vi "get hdf label list swig.vi"(9 "nDevices":i32, 10 "monitor_labels":T1, 11 "file":string) -> (1 "nDevices out":i32, 2 "monitor_labels out":T1, 3 "file out":string, 5 "function return":i32)   [LabVIEW 2019, in "apdm.lvlib"]
doc: "APDM_EXPORT int apdm_get_hdf_label_list_swig(char *file, apdm_monitor_label_t *monitor_labels, int *nDevices);"
uses:
  apdm.lvlib
  Lee Lab/CP FES Walking 2018/Code/Working/LabVIEW/apdm.dll
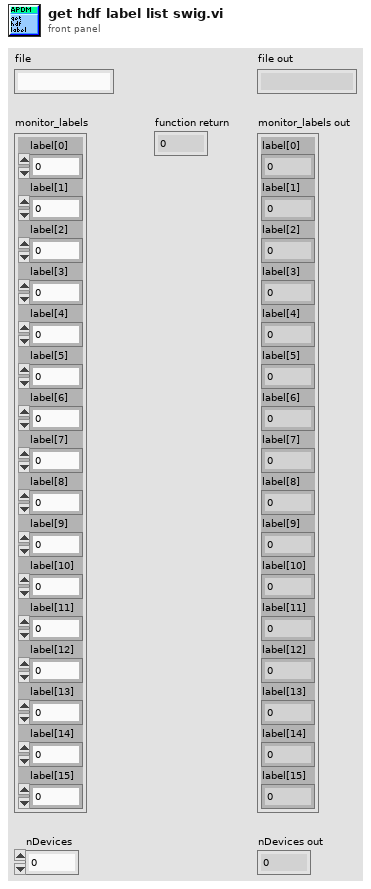
[diagram p1: front panel]
types:
  T1 = cluster{"label[0]":i8, "label[1]":i8, "label[2]":i8, "label[3]":i8, "label[4]":i8, "label[5]":i8, "label[6]":i8, "label[7]":i8, "label[8]":i8, "label[9]":i8, "label[10]":i8, "label[11]":i8, "label[12]":i8, "label[13]":i8, "label[14]":i8, "label[15]":i8}
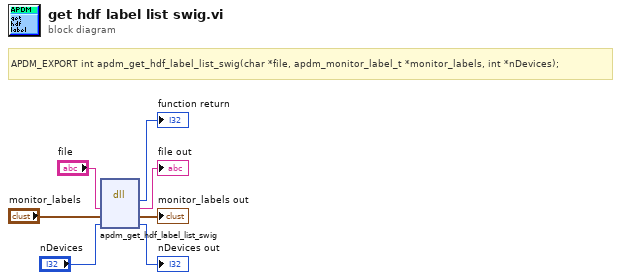
[diagram p0: block diagram]
diagram:
  # "APDM_EXPORT\tint apdm_get_hdf_label_list_swig(char *file, apdm_monitor_label_t *monitor_labels, int *nDevices);"
  n1 = dll-call lib="C:/Users/jfalesi/Dropbox/Lee Lab/CP FES Walking 2018/Code/Working/LabVIEW/apdm.*" fn="apdm_get_hdf_label_list_swig"("file"="file", "monitor_labels"="monitor_labels", "nDevices"="nDevices") -> (→"function return":i32, "file"=→"file out":string, "monitor_labels"=→"monitor_labels out":T1, "nDevices"=→"nDevices out":i32)  [unwired: 3 in, 2 out]
